vi "Change Bold to Strong.vi"(8 "Error In":errorcluster, 11 "Bold Description":string) -> (0 "Error Out":errorcluster, 3 "Strong Description":string)   [LabVIEW 2018, in "Scripts.lvlib"]
uses:
  Scripts.lvlib
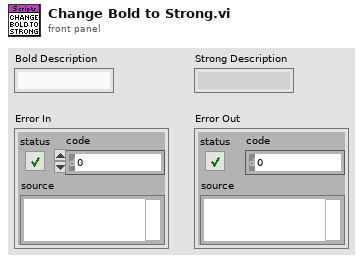
[diagram p1: front panel]
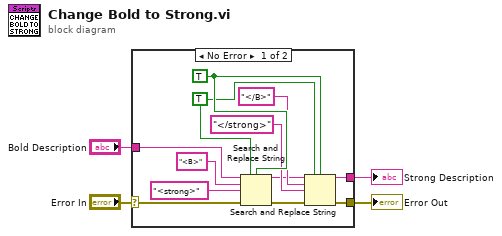
[diagram p0: block diagram]
diagram:
  n1 = case shown="No Error" "Error In" {
    selector: "Error In" -> [w5 w17]
    tunnel: [w11 w17] -> w4
    tunnel: [w10 _] -> w3
    tunnel: "Bold Description" -> [w6 _]
    frame No Error {
      w16 = TRUE ("ignore case? (F)")
      w15 = TRUE ("replace all? (F)")
      n2 = Search and Replace String(replace all?=w15, case sensitive?=w16, input string=w6, search string="<B>", replace string="<strong>" ("replace string (\"\")"), error in=w5) -> (result string=w9:string, error out=w12:errorcluster)  [unwired: 2 in, 2 out]
      n3 = Search and Replace String(replace all?=w15, case sensitive?=w16, input string=w9, search string="</B>", replace string="</strong>" ("replace string (\"\")"), error in=w12) -> (result string=w10:string, error out=w11:errorcluster)  [unwired: 2 in, 2 out]
    }
    frame Error {
    }
  }
  "Error Out" <- w4
  "Strong Description" <- w3
